vi "Current adjust.vi"() -> (0 "Suppressor Voltage":sgl format="%.4f", 1 "Voltage state":bool)   [LabVIEW 2018]
uses:
  Melbourne.llb/energie.gbl
panel:
  out "Output mesure":sgl format="%.2f"
  out "Regul Activated":bool
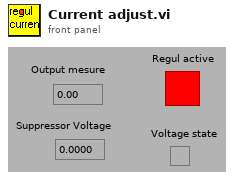
[diagram p1: front panel]
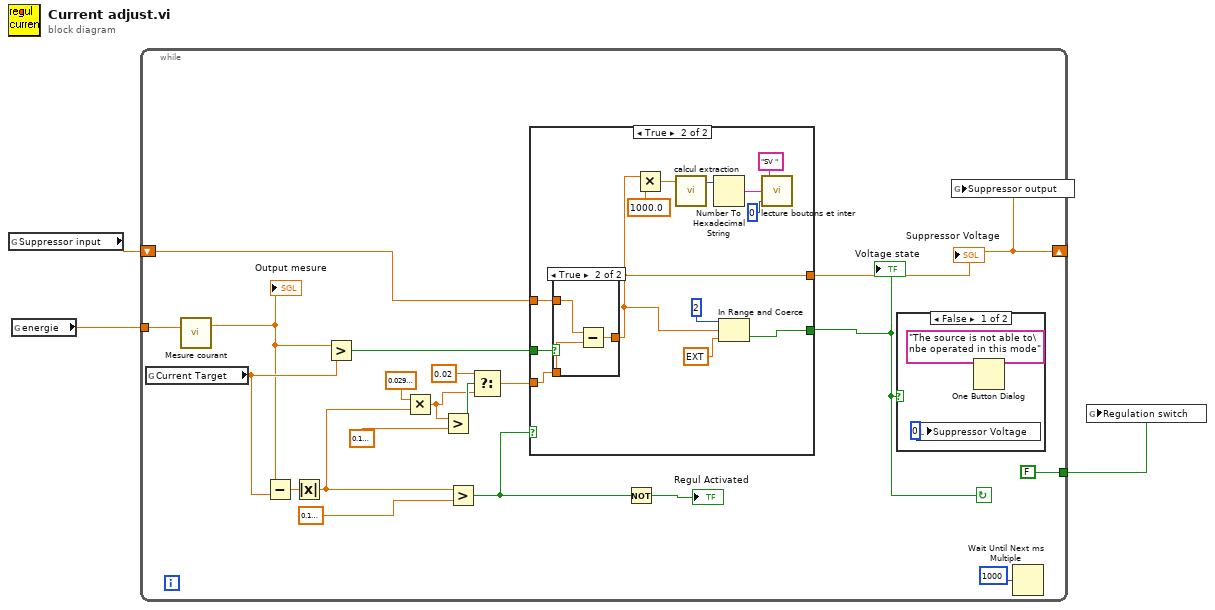
[diagram p0: block diagram]
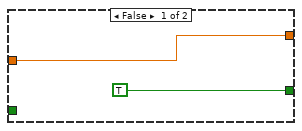
[diagram p3: hidden frame]
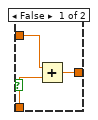
[diagram p4: hidden frame]
diagram:
  n1 = global read "energie.gbl" "Suppressor input"() -> (w2:sgl)
  n2 = global read "energie.gbl" "energie"() -> (w3:sgl)
  n3 = while {
    shift-right: [w18] -> _
    shift-left: w2 -> [w19]
    tunnel: w3 -> [w20]
    tunnel: [FALSE ("Regulation switch")] -> w1
    stop <- w15 continue-if-true
    n4 = global read "energie.gbl" "Current Target"() -> (w14:sgl)
    n5 = call "Mesure courant.vi"("Energy_init"=w20) -> ("Output mesure"=w8:sgl)  [unwired: 1 out]
    "Output mesure" <- w8
    n6 = Subtract(x=w8, y=w14) -> (x-y=w22:sgl)
    n7 = Absolute Value(x=w22) -> (abs(x)=w7:sgl)
    n8 = Greater?(x=w8, y=w14) -> (0:w21:bool)
    n9 = Multiply(x=sgl 0.03, y=w7) -> (x*y=w6:sgl)
    n10 = Greater?(x=w6, y=sgl 0.1) -> (0:w11:bool)
    n11 = Greater?(x=w7, y=sgl 0.1) -> (0:w12:bool)
    n12 = Select(t=0.02, s=w11, f=w6) -> (s? t:f=w9:dbl)
    n13 = case shown="True" w12 {
      tunnel: w19 -> [w27 w40]
      tunnel: [w27 w29] -> w18
      tunnel: w21 -> [_ w39]
      tunnel: w9 -> [_ w38]
      tunnel: [TRUE w28] -> w15
      frame False {
      }
      frame True {
        n14 = case shown="True" w39 {
          tunnel: [w43 w46] -> w29
          tunnel: w40 -> [w42 w45]
          tunnel: w38 -> [w41 w44]
          frame False {
            n15 = Add(x=w42, y=w41) -> (x+y=w43:dbl)
          }
          frame True {
            n16 = Subtract(x=w45, y=w44) -> (x-y=w46:dbl)
          }
        }
        n17 = Multiply(x=w29, y=sgl 1000.0) -> (x*y=w32:dbl)
        n18 = call "calcul extraction.vi"("Entrée extraction"=w32) -> ("Sortie"=w34:i16)
        n19 = Number To Hexadecimal String(2:w34) -> (0:w35:string)  [unwired: 1 in]
        n20 = In Range and Coerce(upper limit=2, x=w29, lower limit=ext 0.0 ("inf")) -> (In Range?=w28:bool)  [unwired: 1 out]
        n21 = call "lecture boutons et inter.vi"("com #"=0, "Ecrit Chaine de carac"=w35, "Entrée Commande"="SV ") -> ()  [unwired: 1 out]
      }
    }
    "Voltage state" <- w15
    "Suppressor Voltage" <- w18
    n22 = Not(x=w12) -> (.not. x?=→"Regul Activated":bool)
    n23 = case shown="False" w15 {
      frame False {
        n24 = local write "Suppressor Voltage"(0) -> ()
        n25 = One Button Dialog(message="The source is not able to\nbe operated in this mode") -> ()  [unwired: 1 in, 1 out]
      }
      frame True {
      }
    }
    n26 = global write "energie.gbl" "Suppressor output"(w18) -> ()
    n27 = Wait Until Next ms Multiple(millisecond multiple=1000) -> ()  [unwired: 1 out]
  }
  n28 = global write "energie.gbl" "Regulation switch"(w1) -> ()
